vi "Load.vi"(0 "Class Loader in":refnum<class "Class Loader.lvclass">, 2 "Loading Method":T1, 5 "Caller Enqueuer":refnum<class "Message Enqueuer.lvclass">, 7 "Reference Class Path":path, 9 "Class Relative Paths Path":path, 11 "error in (no error)":errorcluster) -> (4 "Class Loader out":refnum<class "Class Loader.lvclass">, 15 "error out":errorcluster)   [LabVIEW 2023, in "Class Loader.lvlib" / "Class Loader.lvclass"]
uses:
  Class Loader.lvclass
  Loading Method.ctl
  <vilib>/ActorFramework/Actor/Actor.lvclass/Actor.ctl
  <vilib>/ActorFramework/Message Enqueuer/Message Enqueuer.lvclass/Message Enqueuer.ctl
  <vilib>/ActorFramework/Message Enqueuer/Init from Existing Queue.vi
  Class Loader.lvclass/Class Loader.ctl
  Class Loader Messages/Load Core Parallel Msg/Load Core Parallel Msg.lvclass
  <vilib>/ActorFramework/Actor/Actor.lvclass
  Class Loader Messages/Load Core Sequential Msg/Load Core Sequential Msg.lvclass
  C:/Program Files/National Instruments/LabVIEW 2023/vi.lib/LS Instruments AG/Async Methods Actor/Async Methods Actor/Async Methods Actor/Async Methods Actor.lvclass
  C:/Program Files/National Instruments/LabVIEW 2023/vi.lib/ActorFramework/Actor/Actor.lvclass
  C:/Projects/Shared Libraries/Class Loader/Class Loader/Class Loader/Class Loader.lvclass
  <vilib>/ActorFramework/Message Enqueuer/Message Enqueuer.lvclass
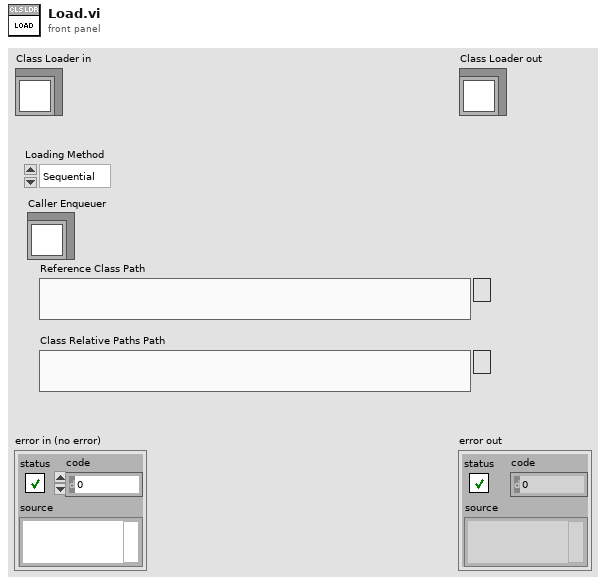
[diagram p1: front panel]
types:
  T1 = typedef "Class Loader.lvlib/Class Loader.lvclass/Loading Method.ctl" = enum16{"Sequential", "Parallel"}
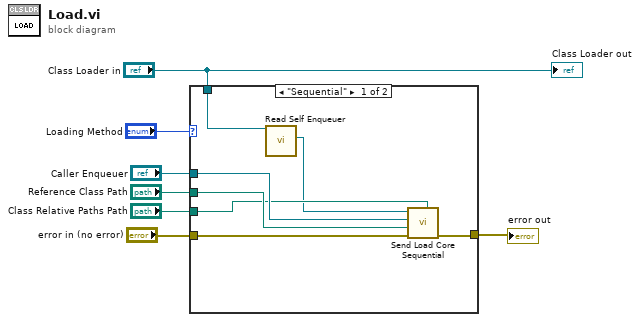
[diagram p0: block diagram]
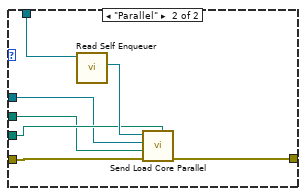
[diagram p2: hidden frame]
diagram:
  n1 = case shown="\"Sequential\"" "Loading Method" {
    tunnel: "Class Loader in" -> [w14 w21]
    tunnel: "error in (no error)" -> [w13 w16]
    tunnel: "Caller Enqueuer" -> [w12 w17]
    tunnel: "Reference Class Path" -> [w11 w18]
    tunnel: "Class Relative Paths Path" -> [w10 w19]
    tunnel: [w9 w15] -> w1
    frame "Sequential" {
      n2 = call <vilib>:"Read Self Enqueuer.vi"("Actor"=w14) -> ("Self Enqueuer"=w8:refnum<class "Message Enqueuer.lvclass">)  [unwired: 10 in]
      n3 = call "Send Load Core Sequential.vi"("Class Relative Paths Path"=w10, "error in (no error)"=w13, "Reference Class Path"=w11, "Caller Enqueuer"=w12, "Message Enqueuer in"=w8) -> ("error out"=w9:errorcluster)  [unwired: 5 in, 1 out]
    }
    frame "Parallel" {
      n4 = call <vilib>:"Read Self Enqueuer.vi"("Actor"=w21) -> ("Self Enqueuer"=w20:refnum<class "Message Enqueuer.lvclass">)  [unwired: 10 in]
      n5 = call "Send Load Core Parallel.vi"("Class Relative Paths Path"=w19, "error in (no error)"=w16, "Reference Class Path"=w18, "Caller Enqueuer"=w17, "Message Enqueuer in"=w20) -> ("error out"=w15:errorcluster)  [unwired: 5 in, 1 out]
    }
  }
  "error out" <- w1
  "Class Loader out" <- "Class Loader in"
